vi "Service ID.vi"(8 "error in (no error)":errorcluster, 11 "HTTPService in":refnum<class "HTTPService.lvclass">) -> (0 "error out":errorcluster, 2 "Service ID":string, 3 "HTTPService out":refnum<class "HTTPService.lvclass">)   [LabVIEW 2020, in "Vecto.lvlib" / "HTTPService.lvclass"]
uses:
  HTTPService.lvclass
  C:/dev/lv20CE/lv-vecto/Vecto/Service/Service.lvclass
  Service/Service.lvclass
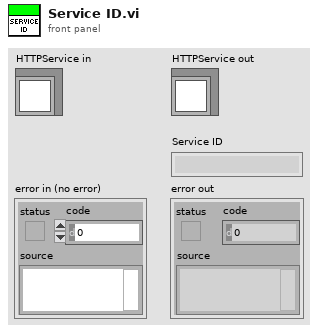
[diagram p1: front panel]
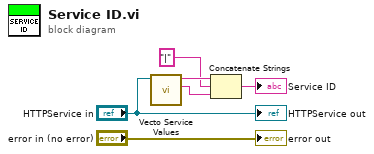
[diagram p0: block diagram]
diagram:
  n1 = call "Vecto Service Values.vi"("Service in"="HTTPService in") -> ("ID"=w3:string, "Type"=w4:string)  [unwired: 9 in]
  n2 = Concatenate Strings(w4, "|", w3) -> (→"Service ID":string)
  "error out" <- "error in (no error)"
  "HTTPService out" <- "HTTPService in"
